vi "Toggle Mute.vi"(7 "Direction":T1, 8 "error in (no error)":errorcluster, 10 "Index":i32, 11 "VMR in":refnum<class "VMR.lvclass">) -> (0 "error out":errorcluster, 2 "Muted":bool, 3 "VMR out":refnum<class "VMR.lvclass">)   [LabVIEW 2022 SP3, in "VMR-Deck.lvlib" / "VMR.lvclass"]
uses:
  VMR.lvclass
  <vilib>/IlluminatedG/IG VoicemeeterRemote API/VoiceMeeterRemote/Direction.ctl
  VMR.lvclass/VMR.ctl
  <vilib>/IlluminatedG/IG VoicemeeterRemote API/VoiceMeeterRemote/VoiceMeeterRemote/VoiceMeeterRemote.lvclass
  <vilib>/IlluminatedG/IG VoicemeeterRemote API/VoiceMeeterRemote/VoiceMeeterRemote.lvlib
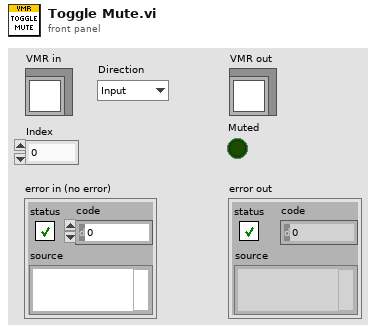
[diagram p1: front panel]
types:
  T1 = typedef "VoiceMeeterRemote.lvlib/Direction.ctl" = enum16{"Input", "Output"}
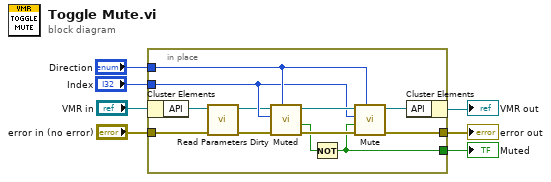
[diagram p0: block diagram]
diagram:
  n1 = in-place {
    in-place-border: "error in (no error)" -> [w19]
    in-place-border: "Direction" -> [w16]
    in-place-border: "Index" -> [w15]
    in-place-border: [w12] -> w2
    in-place-border: [w11] -> w1
    n2 = in-place-cluster #1("VMR in") -> ("API"=w9:refnum<class "VoiceMeeterRemote.lvclass">)
    n3 = call <vilib>:"Read Parameters Dirty.vi"("error in (no error)"=w19, "VoiceMeeterRemote in"=w9) -> ("error out"=w10:errorcluster, "VoiceMeeterRemote out"=w8:refnum<class "VoiceMeeterRemote.lvclass">)  [unwired: 7 in, 1 out]
    n4 = call <vilib>:"Muted.vi"("Direction"=w16, "error in (no error)"=w10, "Index"=w15, "VoiceMeeterRemote in"=w8) -> ("error out"=w18:errorcluster, "Muted?"=w14:bool, "VoiceMeeterRemote out"=w17:refnum<class "VoiceMeeterRemote.lvclass">)  [unwired: 5 in]
    n5 = Not(x=w14) -> (.not. x?=w11:bool)
    n6 = call <vilib>:"Mute.vi"("Direction"=w16, "error in (no error)"=w18, "Mute? (T)"=w11, "Index"=w15, "VoiceMeeterRemote in"=w17) -> ("error out"=w12:errorcluster, "VoiceMeeterRemote out"=w13:refnum<class "VoiceMeeterRemote.lvclass">)  [unwired: 5 in]
    n7 = in-place-cluster #1("API"=w13) -> (→"VMR out":refnum<class "VMR.lvclass">)
  }
  "error out" <- w2
  "Muted" <- w1
